vi "Harris_4th_Exercise0_12-1-16.vi"   [LabVIEW 2014, in "Harris_MacMaster_4th_LEGORobotics_11-29-16.lvrbt"]
uses:
  Harris_MacMaster_4th_LEGORobotics_11-29-16.lvrbt
  <vilib>/NXT/Dual Mode Library/Display/drawText.vi
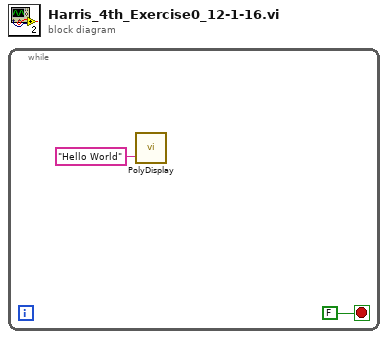
[diagram p0: block diagram]
diagram:
  n1 = while {
    stop <- FALSE stop-if-true
    n2 = call-poly <vilib>:"PolyDisplay.vi"("Text"="Hello World") -> ()  [unwired: 3 in, 1 out]
  }
